vi "Global Variables.vi"() -> ()   [LabVIEW 2021, in "XNET-CAN-Signal-Logger.lvlib"]
uses:
  XNET-CAN-Signal-Logger.lvlib
panel:
  out "Signal Data":variant[](array[variant])
  in  "Error Queue Name":string="Error Queue"
  out "Signal Units":variant[](array[variant])
  out "Signal Names":variant[](array[variant])
  out "Global Stop":bool
  in  "Log File Group Name":string="Log"
  in  "TDMS Data Queue Name":string="TDMS Data Queue"
  # "Constants"
  # "Variables"
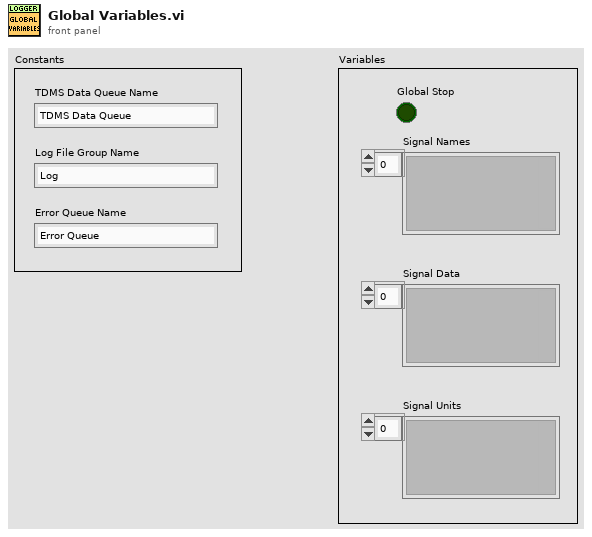
[diagram p1: front panel]
diagram:
